vi "CaseStructure - Get Group Seperator Case Index.vi"(8 "error in (no error)":errorcluster, 10 "Group Name":string, 11 "CaseStructure in":refnum<vi>) -> (0 "error out":errorcluster, 2 "Numeric":i32, 3 "CaseStructure out":refnum<vi>)   [LabVIEW 2017, in "csmHelper-CaseStructure.lvlib"]
doc: "-- <b>输入控件</b> --\n\n- <b>Group Name</b>:\n\n- <b>CaseStructure in</b>:\n\n-- <b>输出控件</b> --\n\n- <b>Numeric</b>:\n\n- <b>CaseStructure out</b>:"
uses:
  csmHelper-CaseStructure.lvlib
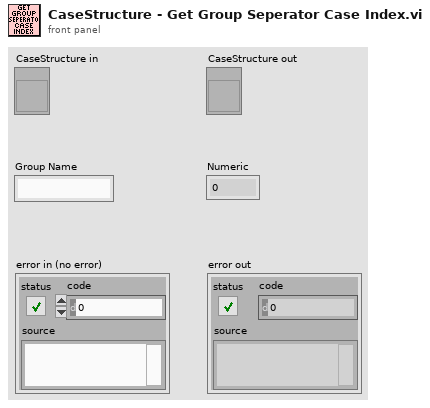
[diagram p1: front panel]
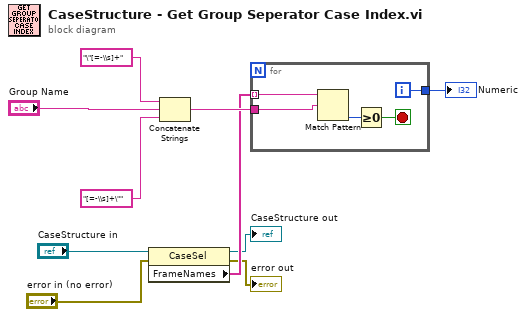
[diagram p0: block diagram]
diagram:
  n1 = property class="CaseSel"(reference="CaseStructure in", error in="error in (no error)") -> (reference out=→"CaseStructure out":refnum<vi>, error out=→"error out":errorcluster, "FrameNames"=w6:string[])
  n2 = Concatenate Strings("\"[=-\\s]+" ("regular expression"), "Group Name", "[=-\\s]+\"" ("regular expression")) -> (w10:string)
  n3 = for {
    tunnel: w6 -> [w15] mode=indexing
    tunnel: w10 -> [w13]
    tunnel: [w14] -> w7
    i -> [w14]
    stop <- w11 stop-if-true
    n4 = Match Pattern(string=w15, regular expression=w13) -> (offset past match=w12:i32)  [unwired: 1 in, 3 out]
    n5 = Greater Or Equal To 0?(x=w12) -> (x >= 0?=w11:bool)
  }
  "Numeric" <- w7
